vi "Part Features.vi"(8 "error in (no error)":errorcluster, 9 "Feature Names":string[](array[string]), 10 "Part Name":string, 11 "FlexWorktable in":refnum<class "FlexWorktable.lvclass">) -> (0 "error out":errorcluster, 2 "Features":T1(array[cluster]), 3 "FlexWorktable out":refnum<class "FlexWorktable.lvclass">)   [LabVIEW 2017, in "FlexWorktable.lvclass"]
uses:
  FlexWorktable.lvclass
  Vec3d Class/Vec3d.lvclass
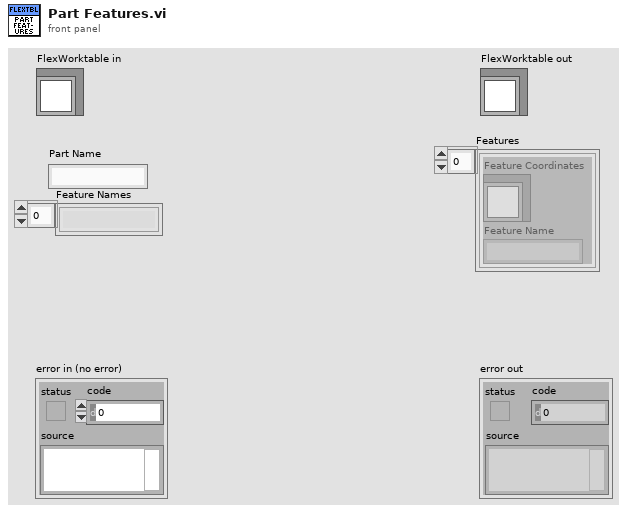
[diagram p1: front panel]
types:
  T1 = cluster{"Feature Coordinates":refnum<class "Vec3d.lvclass">, "Feature Name":string}[]
  T2 = cluster{"Feature Coordinates":refnum<class "Vec3d.lvclass">, "Feature Name":string}
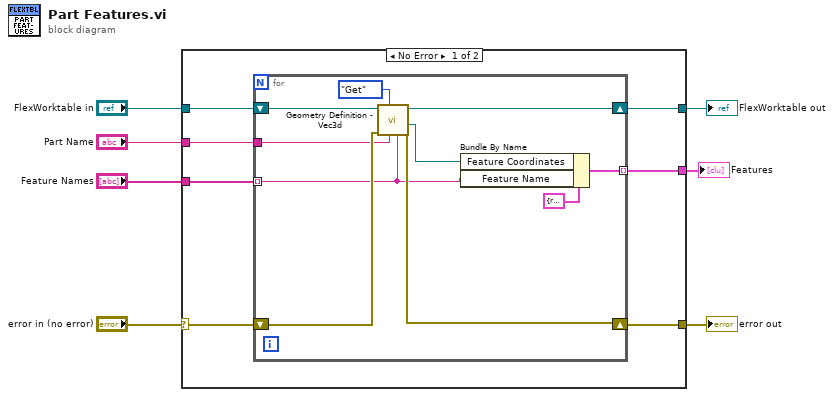
[diagram p0: block diagram]
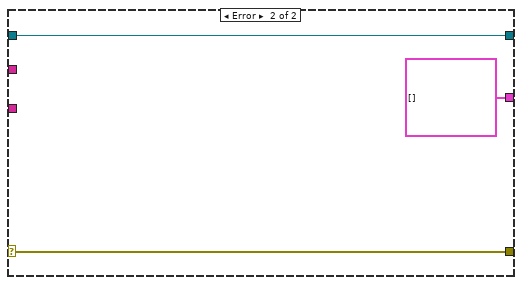
[diagram p2: hidden frame]
diagram:
  n1 = case shown="No Error" "error in (no error)" {
    selector: "error in (no error)" -> [w11 w27]
    tunnel: [w10 w27] -> w6
    tunnel: [w8 w26] -> w4
    tunnel: "FlexWorktable in" -> [w14 w26]
    tunnel: "Part Name" -> [w13 _]
    tunnel: "Feature Names" -> [w12 _]
    tunnel: [w9 T1 []] -> w1
    frame No Error {
      n2 = for {
        tunnel: w13 -> [w17]
        tunnel: w12 -> [w15] mode=indexing
        shift-right: [w18] -> w10
        shift-left: w11 -> [w21]
        tunnel: [w16] -> w9 mode=indexing
        shift-right: [w22] -> w8
        shift-left: w14 -> [w24]
        n3 = call-dynamic "Geometry Definition - Vec3d.vi"("Feature Name"=w15, "Part Type"=w17, "Get/Set"=enum16{"Get", "Set"}."Get", "error in (no error)"=w21, "FlexWorktable in"=w24) -> ("error out"=w18:errorcluster, "Geometry Definition out"=w19:refnum<class "Vec3d.lvclass">, "FlexWorktable out"=w22:refnum<class "FlexWorktable.lvclass">)  [unwired: 4 in]
        n4 = Bundle By Name(cluster=T2 {"Feature Coordinates"=refnum, "Feature Name"=""} ("Feature Description"), "Feature Coordinates"=w19, "Feature Name"=w15) -> (w16:T2)
      }
    }
    frame Error {
    }
  }
  "error out" <- w6
  "FlexWorktable out" <- w4
  "Features" <- w1
